vi "Write trackID.vi"(8 "error in (no error)":errorcluster, 10 "trackID":dbl, 11 "GWTargetPositionParameters in":refnum<class "GWTargetPositionParameters.lvclass">) -> (0 "error out":errorcluster, 3 "GWTargetPositionParameters out":refnum<class "GWTargetPositionParameters.lvclass">)   [LabVIEW 2022 SP3, in "TCSDataDefinitions.lvlib" / "TCSGuiderStatus.lvlib" / "GWTargetPositionParameters.lvclass"]
uses:
  GWTargetPositionParameters.lvclass
  GWTargetPositionParameters.lvclass/GWTargetPositionParameters.ctl
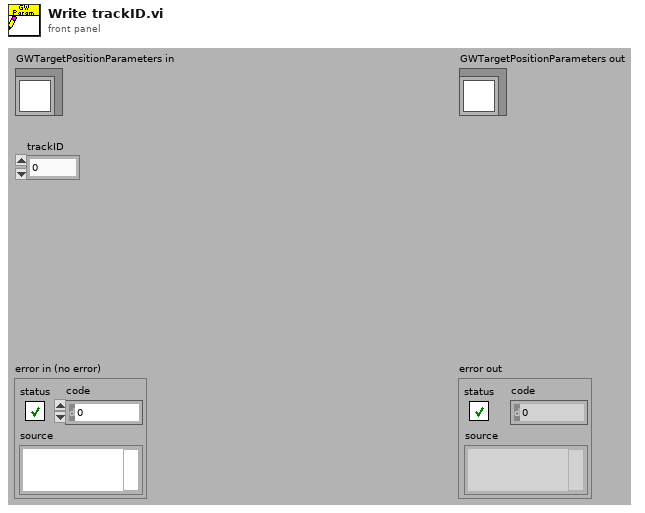
[diagram p1: front panel]
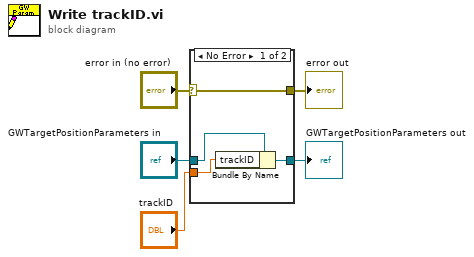
[diagram p0: block diagram]
diagram:
  n1 = case shown="No Error" "error in (no error)" {
    selector: "error in (no error)" -> [w9 w10]
    tunnel: [w9 w10] -> w4
    tunnel: [w7 w11] -> w2
    tunnel: "GWTargetPositionParameters in" -> [w8 w11]
    tunnel: "trackID" -> [w6 _]
    frame No Error {
      n2 = Bundle By Name(cluster=w8, "trackID"=w6) -> (w7:refnum<class "GWTargetPositionParameters.lvclass">)
    }
    frame Error {
    }
  }
  "error out" <- w4
  "GWTargetPositionParameters out" <- w2
